vi "In Progress 2.vi"() -> ()   [LabVIEW 2013]
uses:
  <vilib>/Rock Robotics/WPI/Solenoid/WPI_SolenoidValue.ctl
panel:
  out "Value":T1
  out "Value":T1
  in  "Speed 2":dbl
  in  "Low Change 2":dbl
  in  "High Change 2":dbl
  out "Value":T1
  out "Value":T1
  in  "Shift?":bool
  in  "Current shift Logic":bool
  in  "High Change":dbl
  in  "Low Change":dbl
  in  "Speed":dbl
  in  "Speed":dbl
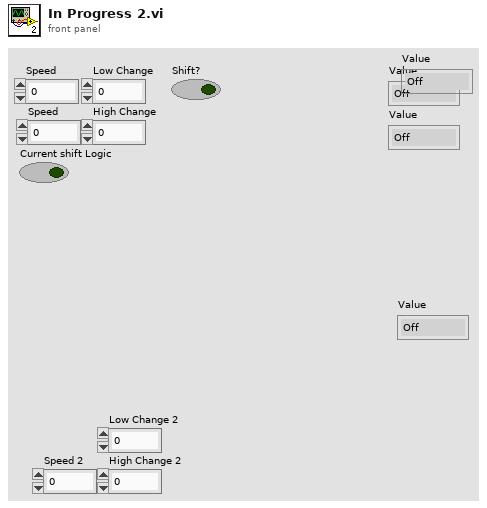
[diagram p1: front panel]
types:
  T1 = typedef "WPI_SolenoidValue.ctl" = enum16{"Off", "On", "Forward", "Reverse"}
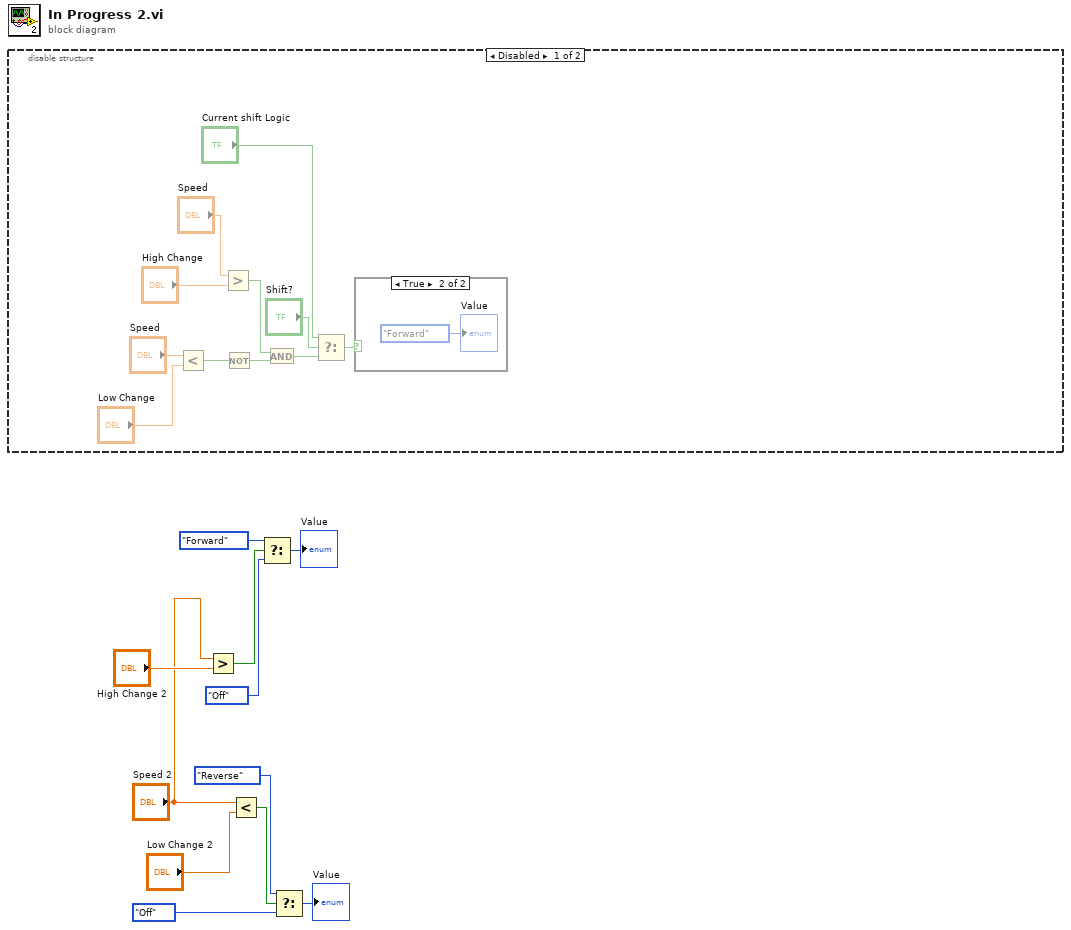
[diagram p0: block diagram]
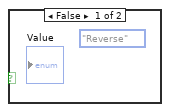
[diagram p2: hidden frame]
diagram:
  n1 = disable-structure shown="Disabled" {
    frame Disabled {
      n2 = Less?(x="Speed", y="Low Change") -> (x < y?=w18:bool)
      n3 = Greater?(x="Speed", y="High Change") -> (0:w17:bool)
      n4 = Not(x=w18) -> (.not. x?=w16:bool)
      n5 = And(x=w17, y=w16) -> (x .and. y?=w12:bool)
      n6 = Select(t="Current shift Logic", s="Shift?", f=w12) -> (s? t:f=w14:bool)
      n7 = case shown="True" w14 {
        frame False {
          (unwired) WPI_SolenoidValue."Reverse" ("Value")
        }
        frame True {
          "Value" <- WPI_SolenoidValue."Forward" ("Value")
        }
      }
    }
    frame Enabled {
    }
  }
  n8 = Greater?(x="Speed 2", y="High Change 2") -> (0:w9:bool)
  n9 = Less?(x="Speed 2", y="Low Change 2") -> (x < y?=w2:bool)
  n10 = Select(t=WPI_SolenoidValue."Forward" ("Value"), s=w9, f=WPI_SolenoidValue."Off") -> (s? t:f=→"Value":T1)
  n11 = Select(t=WPI_SolenoidValue."Reverse" ("Value"), s=w2, f=WPI_SolenoidValue."Off") -> (s? t:f=→"Value":T1)
